vi "Update G.vi"(8 "error in (no error)":errorcluster, 10 "SLAM In":T3, 11 "New LM's In":T2(array[cluster])) -> (0 "error out":errorcluster, 2 "SLAM Out":T3, 3 "New LM's Out":T2(array[cluster]))   [LabVIEW 2009]
uses:
  <vilib>/Analysis/Matrix/Datatypes/RealMatrix.ctl
  Controls/SLAM.ctl
  <vilib>/Analysis/Matrix/NI_Matrix.lvlib
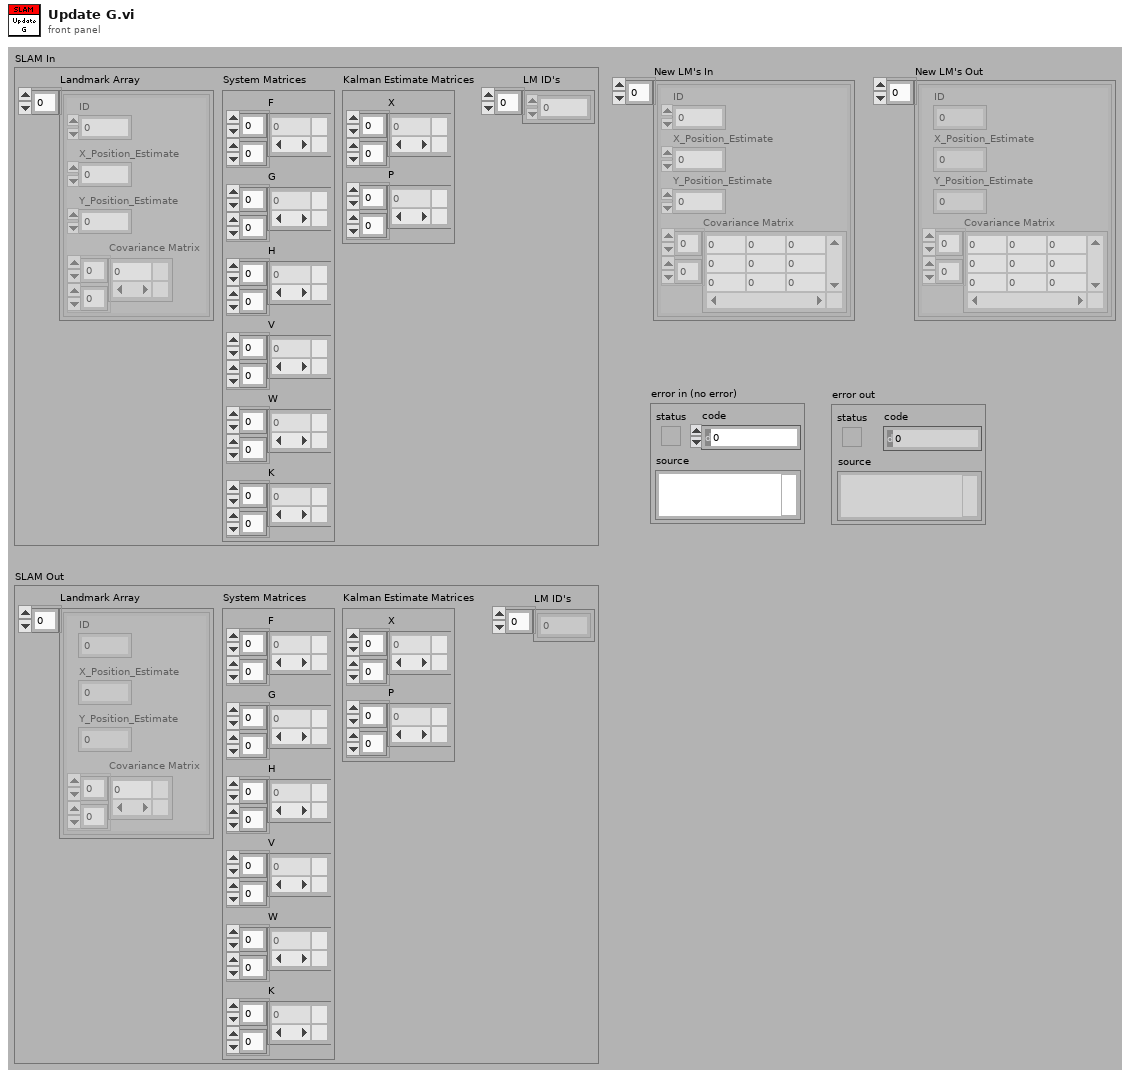
[diagram p1: front panel]
types:
  T1 = typedef "NI_Matrix.lvlib/RealMatrix.ctl" = dbl[][]
  T2 = cluster{"ID":dbl, "X_Position_Estimate":dbl, "Y_Position_Estimate":dbl, "Covariance Matrix":T1}[]
  T3 = typedef "SLAM.ctl" = cluster{"Landmark Array":cluster{"ID":dbl, "X_Position_Estimate":dbl, "Y_Position_Estimate":dbl, "Covariance Matrix":T1}[], "System Matrices":cluster{"F":T1, "G":T1, "H":T1, "V":T1, "W":T1, "K":T1}, "Kalman Estimate Matrices":cluster{"X":T1, "P":T1}, "LM ID's":dbl[]}
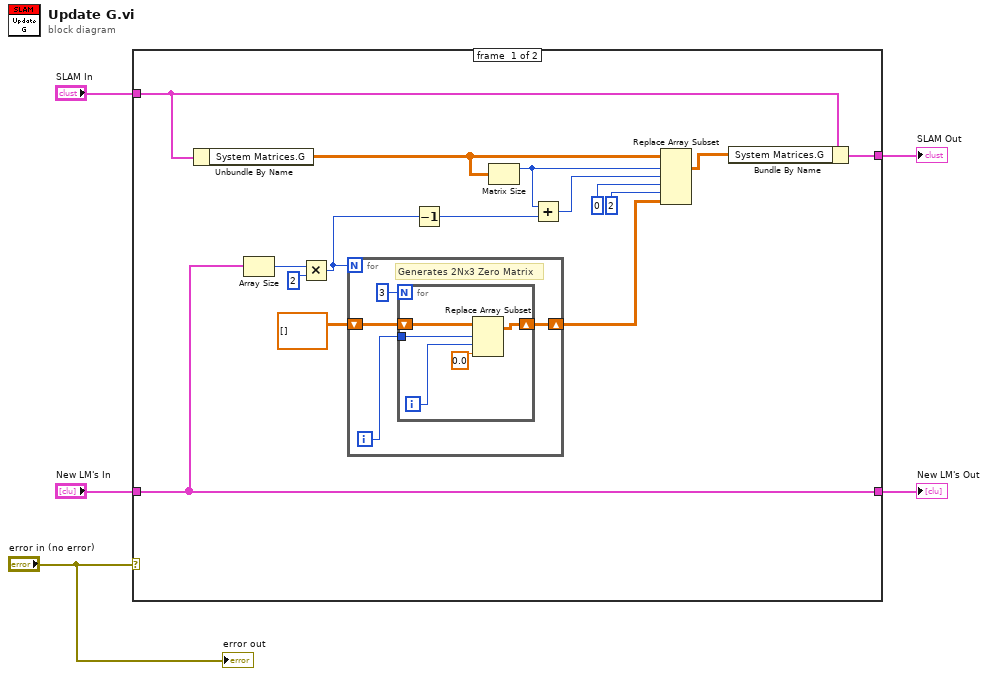
[diagram p0: block diagram]
diagram:
  n1 = case shown="No Error" "error in (no error)" {
    tunnel: "SLAM In" -> [w19 w30]
    tunnel: "New LM's In" -> [w13 w31]
    tunnel: [w14 w30] -> w3
    tunnel: [w13 w31] -> w2
    frame #0 {
      n2 = Unbundle By Name(w19) -> ("System Matrices.G"=w10:T1)
      n3 = Array Size(array=w13) -> (size(s)=w8:i32)
      n4 = Multiply(x=w8, y=2) -> (x*y=w6:i32)
      n5 = for {
        N: w6 -> [_]
        shift-right: [w22] -> w16
        shift-left: T1 [] ("matrix") -> [w24]
        i -> [w23]
        # "Generates 2Nx3 Zero Matrix"
        n6 = for {
          N: 3 -> [_]
          shift-right: [w28] -> w22
          shift-left: w24 -> [w29]
          tunnel: w23 -> [w27]
          i -> [w26]
          n7 = Replace Array Subset(array=w29, new element=0.0 ("new element/submatrix"), index (row)=w27, index (col)=w26) -> (w28:T1)
        }
      }
      n8 = Decrement(x=w6) -> (x-1=w15:i32)
      n9 = Matrix Size(0:w10) -> (1:w18:i32)  [unwired: 1 out]
      n10 = Add(x=w18, y=w15) -> (x+y=w17:i32)
      n11 = Replace Array Subset(array=w10, new element=w16, index (dim 0)=w18, index (dim 1)=w17, index (dim 2)=0 ("column 1"), index (dim 3)=2 ("column 1")) -> (w9:T1)
      n12 = Bundle By Name(cluster=w19, "System Matrices.G"=w9) -> (w14:T3)
    }
    frame #1 {
    }
  }
  "New LM's Out" <- w2
  "SLAM Out" <- w3
  "error out" <- "error in (no error)"
